vi "pulse_output.vi"(8 "error in":errorcluster, 9 "low times":dbl format="%#_13g", 10 "pulse number":i32, 11 "high times":dbl format="%#_13g") -> (0 "error out":errorcluster)   [LabVIEW 2013]
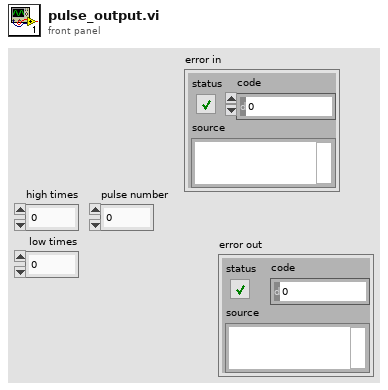
[diagram p1: front panel]
types:
  T1 = cluster{"high times":dbl, "low times":dbl, "pulse number":i32, "cmd":string, "status":string}
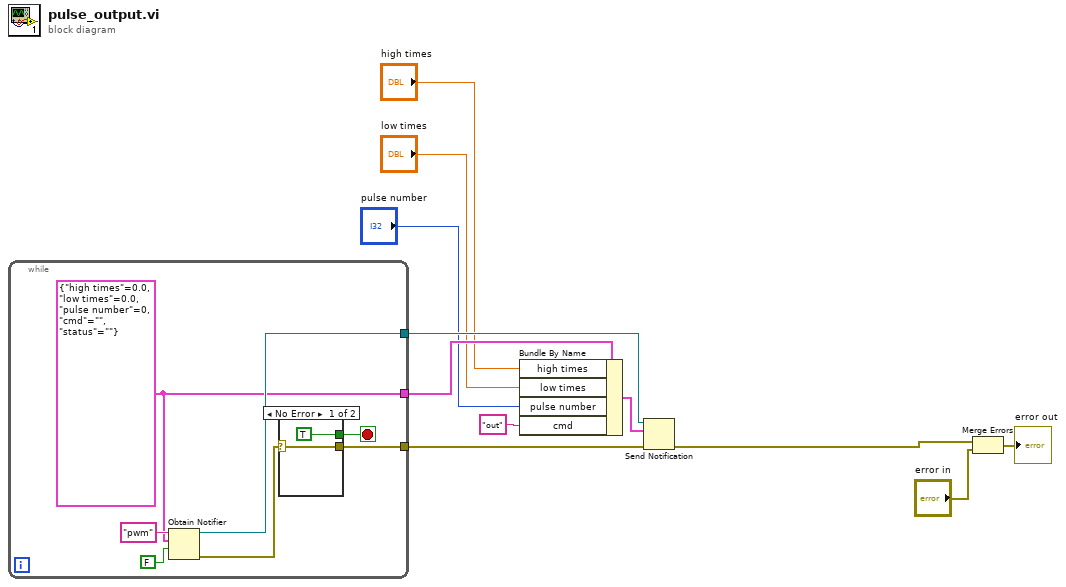
[diagram p0: block diagram]
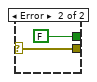
[diagram p2: hidden frame]
diagram:
  n1 = while {
    tunnel: [w16] -> w11
    tunnel: [w12] -> w10
    tunnel: [w15] -> w9
    stop <- w13 stop-if-true
    w15 = T1 {"high times"=0.0, "low times"=0.0, "pulse number"=0, "cmd"="", "status"=""}
    n2 = Obtain Notifier(name (unnamed)="pwm", notification data type=w15, create if not found? (T)=FALSE) -> (notifier out=w16:refnum<notifier>, error out=w14:errorcluster)  [unwired: 1 in, 1 out]
    n3 = case shown="No Error" w14 {
      selector: w14 -> [w19 w21]
      tunnel: [TRUE FALSE] -> w13
      tunnel: [w19 w21] -> w12
      frame No Error {
      }
      frame Error {
      }
    }
  }
  n4 = Bundle By Name(cluster=w9, "high times"="high times", "low times"="low times", "pulse number"="pulse number", "cmd"="out") -> (w4:T1)
  n5 = Send Notification(notification=w4, notifier=w11, error in (no error)=w10) -> (error out=w2:errorcluster)  [unwired: 1 out]
  n6 = Merge Errors(w2, "error in") -> (→"error out":errorcluster)
